vi "Exclude and Tidy Library File.vi"(6 "Exclude dependent packed libraries (T)":bool=TRUE, 8 "error in (no error)":errorcluster, 11 "NI_AB_API_PPL in":refnum<class "NI_AB_API_PPL.lvclass">) -> (0 "error out":errorcluster, 3 "NI_AB_API_PPL out":refnum<class "NI_AB_API_PPL.lvclass">)   [LabVIEW 2019]
uses:
  <vilib>/AppBuilder/AB_API/PPL/NI_AB_API_PPL.lvclass
  <vilib>/AppBuilder/AB_API/common/AB_API Primary Exclusions.ctl
  <vilib>/AppBuilder/AB_API/common/AB_API Path Exclusions.ctl
  <vilib>/AppBuilder/AB_API/DPPL/NI_AB_API_DPPL.lvclass
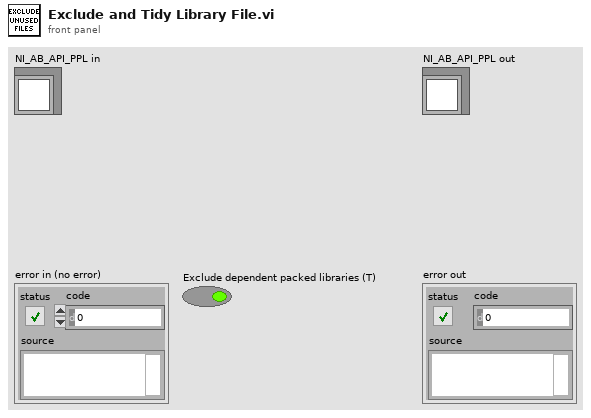
[diagram p1: front panel]
types:
  T1 = typedef "AB_API Primary Exclusions.ctl" = cluster{"Disconnect type definitions":bool, "Remove unused polymorphic VI instances":bool, "Remove unused members of project libraries":bool, "Modify project library file after removing unused members":bool}
  T2 = typedef "AB_API Path Exclusions.ctl" = cluster{"Exclude files from vi.lib":bool, "Exclude files from instr.lib":bool, "Exclude files from user.lib":bool}
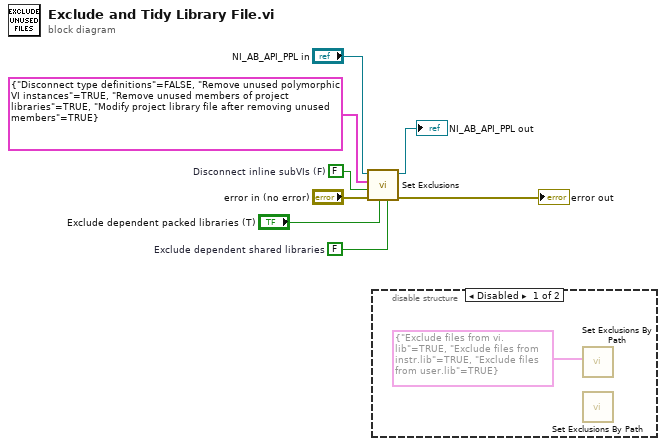
[diagram p0: block diagram]
diagram:
  w4 = FALSE  # Disconnect inline subVIs (F)
  w2 = FALSE  # Exclude dependent shared libraries
  n1 = call-dynamic "Set Exclusions.vi"("Exclude dependent shared libraries"=w2, "Exclude dependent packed libraries"="Exclude dependent packed libraries (T)", "error in (no error)"="error in (no error)", "Disconnect inline subVIs (F)"=w4, "Exclusions"=T1 {"Disconnect type definitions"=FALSE, "Remove unused polymorphic VI instances"=TRUE, "Remove unused members of project libraries"=TRUE, "Modify project library file after removing unused members"=TRUE}, "PPL in"="NI_AB_API_PPL in") -> ("error out"=→"error out":errorcluster, "PPL out"=→"NI_AB_API_PPL out":refnum<class "NI_AB_API_PPL.lvclass">)  [unwired: 4 in]
  n2 = disable-structure shown="Disabled" {
    frame Disabled {
      n3 = call-dynamic "Set Exclusions By Path.vi"("Path exclusions"=T2 {"Exclude files from vi.lib"=TRUE, "Exclude files from instr.lib"=TRUE, "Exclude files from user.lib"=TRUE}) -> ()  [unwired: 9 in, 2 out]
      n4 = call-dynamic "Set Exclusions By Path.vi"() -> ()  [unwired: 10 in, 2 out]
    }
    frame Enabled {
    }
  }
